vi "SetPosition.vi"(1 "Current Position (µm)":cluster{"x":dbl, "y":dbl, "z":dbl} {"z" format="%.2f"; "y" format="%.2f"; "x" format="%.2f"}) -> (0 "error out":errorcluster)   [LabVIEW 2009]
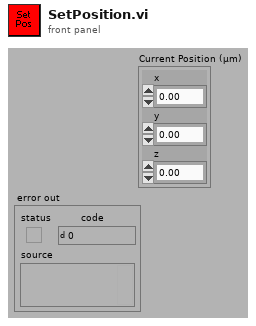
[diagram p1: front panel]
types:
  T1 = enum16{"Get Type", "Set Type", "GetStageInit", "GetWriteStageSetting", "GetInitializeStageOutput", "GetSetAxisPosition", "GetSetPos"}
  T2 = typedef "StageType.ctt" = enum16{"PI analogue", "PI 712 TCP/IP", "Märzhäuser", "PI analogue step", "PI 712 USB"}
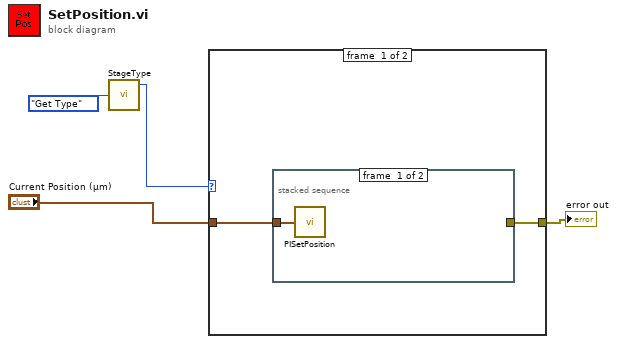
[diagram p0: block diagram]
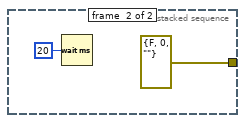
[diagram p2: hidden frame]
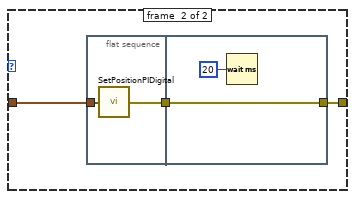
[diagram p3: hidden frame]
diagram:
  n1 = call "StageType.vi"("Function"=T1."Get Type") -> ("Stage Type (output)"=w2:T2)  [unwired: 2 in, 2 out]
  n2 = case shown="\"PI 712 TCP/IP\", \"PI 712 USB\"" w2 {
    tunnel: "Current Position (µm)" -> [w6 w12]
    tunnel: [w5 w11] -> w1
    frame #0 {
      n3 = stacked-sequence {
        tunnel: w6 -> [w7 _]
        tunnel: [_ errorcluster {"status"=FALSE, "code"=0, "source"=""} ("error out")] -> w5
        frame #0 {
          n4 = call "PISetPosition.vi"("Current Position (µm)"=w7) -> ()
        }
        frame #1 {
          n5 = Wait (ms)(milliseconds to wait=u32 20) -> ()  [unwired: 1 out]
        }
      }
    }
    frame #1 {
      n6 = flat-sequence {
        tunnel: w12 -> [w14]
        tunnel: [w13] -> w10
        tunnel: [w16] -> w11
        tunnel: w10 -> [w16]
        frame #0 {
          n7 = call "SetPositionPIDigital.vi"("Current Position (µm)"=w14) -> ("error out"=w13:errorcluster)
        }
        frame #1 {
          n8 = Wait (ms)(milliseconds to wait=u32 20) -> ()  [unwired: 1 out]
        }
      }
    }
  }
  "error out" <- w1
